vi "Charging_Find IPG MICS IDs.vi"(6 "error in":errorcluster, 8 "MICS_Config_In":T1={"ConfigFlags"=0, "ImplantID"=0, "CompanyID"=187, "Normal_Comm"={"RF_Channel"=4, "UserData"=0, "TX_Mod"=0, "RX_Mod"=0, "RX_BlockSize"=15, "BlockPerPack"=31, "TX_BlockSize"=15}, "Emerg_Comm"={"RF_Channel"=4, "UserData"=0, "TX_Mod"=0, "RX_Mod"=0, "TX_BlockSize"=15, "BlockPerPack"=31, "RX_BlockSize"=15}, "ImplantRev"=4, "245TX_PowerCal"=0, "245TX_Power"=10, "CCA_RSSI_Thresholds"={"ch0"=2650, "ch1"=2650, "ch2"=2650, "ch3"=2650, "ch4"=2650, "ch5"=2650, "ch6"=2650, "ch7"=2650, "ch8"=2650, "ch9"=2650}} {"ImplantID" format="%04x"; "CompanyID" format="%.0x"; "Normal_Comm"."RF_Channel" items=["0", "1", "2", "3", "4", "5", "6", "7", "8", "9"]; "Normal_Comm"."UserData" items=["0 - 000"=0, "1 - 001"=16, "2 - 010"=32, "3 - 011"=48, "4 - 100"=64, "5 - 101"=80, "6 - 110"=96, "7 - 111"=112]; "Normal_Comm"."TX_Mod" items=["2FSK-FB"=0, "2FSK"=2, "4FSK"=3]; "Normal_Comm"."RX_Mod" items=["2FSK-FB"=0, "2FSK"=8, "4FSK"=12]; "Normal_Comm"."RX_BlockSize" items=["2"=2, "3"=3, "4"=4, "5"=5, "6"=6, "7"=7, "8"=8, "9"=9, "10"=10, "11"=11, "12"=12, "13"=13, "14"=14, "15"=15, "16"=16, "17"=17, "18"=18, "19"=19, "20"=20, "21"=21, "22"=22, "23"=23, "24"=24, "25"=25, "26"=26, "27"=27, "28"=28, "29"=29, "30"=30, "31"=31]; "Normal_Comm"."BlockPerPack" items=["1"=1, "2"=2, "3"=3, "4"=4, "5"=5, "6"=6, "7"=7, "8"=8, "9"=9, "10"=10, "11"=11, "12"=12, "13"=13, "14"=14, "15"=15, "16"=16, "17"=17, "18"=18, "19"=19, "20"=20, "21"=21, "22"=22, "23"=23, "24"=24, "25"=25, "26"=26, "27"=27, "28"=28, "29"=29, "30"=30, "31"=31]; "Normal_Comm"."TX_BlockSize" items=["2"=2, "3"=3, "4"=4, "5"=5, "6"=6, "7"=7, "8"=8, "9"=9, "10"=10, "11"=11, "12"=12, "13"=13, "14"=14, "15"=15, "16"=16, "17"=17, "18"=18, "19"=19, "20"=20, "21"=21, "22"=22, "23"=23, "24"=24, "25"=25, "26"=26, "27"=27, "28"=28, "29"=29, "30"=30, "31"=31]; "Emerg_Comm"."RF_Channel" items=["0", "1", "2", "3", "4", "5", "6", "7", "8", "9"]; "Emerg_Comm"."UserData" items=["0 - 000"=0, "1 - 001"=16, "2 - 010"=32, "3 - 011"=48, "4 - 100"=64, "5 - 101"=80, "6 - 110"=96, "7 - 111"=112]; "Emerg_Comm"."TX_Mod" items=["2FSK-FB"=0, "2FSK"=2, "4FSK"=3]; "Emerg_Comm"."RX_Mod" items=["2FSK-FB"=0, "2FSK"=8, "4FSK"=12]; "Emerg_Comm"."TX_BlockSize" items=["2"=2, "3"=3, "4"=4, "5"=5, "6"=6, "7"=7, "8"=8, "9"=9, "10"=10, "11"=11, "12"=12, "13"=13, "14"=14, "15"=15, "16"=16, "17"=17, "18"=18, "19"=19, "20"=20, "21"=21, "22"=22, "23"=23, "24"=24, "25"=25, "26"=26, "27"=27, "28"=28, "29"=29, "30"=30, "31"=31]; "Emerg_Comm"."BlockPerPack" items=["1"=1, "2"=2, "3"=3, "4"=4, "5"=5, "6"=6, "7"=7, "8"=8, "9"=9, "10"=10, "11"=11, "12"=12, "13"=13, "14"=14, "15"=15, "16"=16, "17"=17, "18"=18, "19"=19, "20"=20, "21"=21, "22"=22, "23"=23, "24"=24, "25"=25, "26"=26, "27"=27, "28"=28, "29"=29, "30"=30, "31"=31]; "Emerg_Comm"."RX_BlockSize" items=["2"=2, "3"=3, "4"=4, "5"=5, "6"=6, "7"=7, "8"=8, "9"=9, "10"=10, "11"=11, "12"=12, "13"=13, "14"=14, "15"=15, "16"=16, "17"=17, "18"=18, "19"=19, "20"=20, "21"=21, "22"=22, "23"=23, "24"=24, "25"=25, "26"=26, "27"=27, "28"=28, "29"=29, "30"=30, "31"=31]; "ImplantRev" items=["ZL70100"=0, "ZL70101"=1, "ZL70102"=4]; "245TX_PowerCal" items=["-29"=-29, "-4"=-4, "-2"=-2, "0"=0, "2"=2, "4"=4, "6"=6, "8"=8, "10"=10, "12"=12, "14"=14, "16"=16, "18"=18, "20"=20, "22"=22, "24"=24, "26"=26, "27"=27]; "245TX_Power" items=["-29"=-29, "-4"=-4, "-2"=-2, "0"=0, "2"=2, "4"=4, "6"=6, "8"=8, "10"=10, "12"=12, "14"=14, "16"=16, "18"=18, "20"=20, "22"=22, "24"=24, "26"=26, "27"=27]}, 9 "MICS COM port":refnum<visa-resource-name>="COM11") -> (0 "error out":errorcluster {"code" format="%.0x"}, 3 "detected MICS IDs":u32[](array[numeric]))   [LabVIEW 2020]
doc: "This function searches for IPGs MIC IDs. The MICS Setup and MICS Config operations are performed before searching for the MICS IDs."
panel:
  in  "Max # of Attempts to Find Device":i32=3
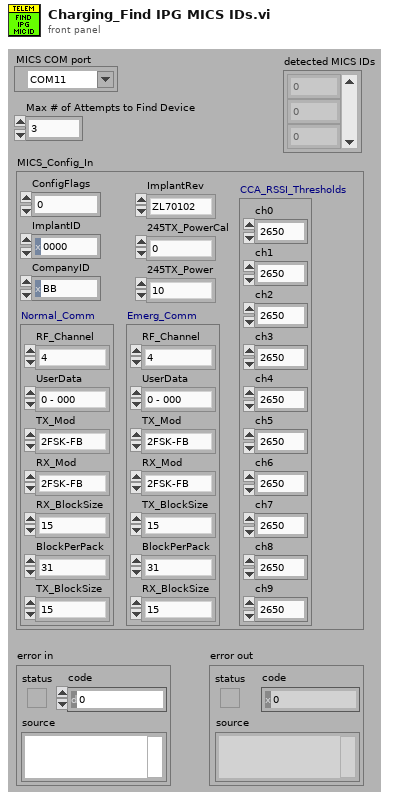
[diagram p1: front panel]
types:
  T1 = cluster{"ConfigFlags":u8, "ImplantID":u32, "CompanyID":u8, "Normal_Comm":cluster{"RF_Channel":u8, "UserData":u8, "TX_Mod":u8, "RX_Mod":u8, "RX_BlockSize":u8, "BlockPerPack":u8, "TX_BlockSize":u8}, "Emerg_Comm":cluster{"RF_Channel":u8, "UserData":u8, "TX_Mod":u8, "RX_Mod":u8, "TX_BlockSize":u8, "BlockPerPack":u8, "RX_BlockSize":u8}, "ImplantRev":u8, "245TX_PowerCal":i8, "245TX_Power":i8, "CCA_RSSI_Thresholds":cluster{"ch0":u16, "ch1":u16, "ch2":u16, "ch3":u16, "ch4":u16, "ch5":u16, "ch6":u16, "ch7":u16, "ch8":u16, "ch9":u16}}
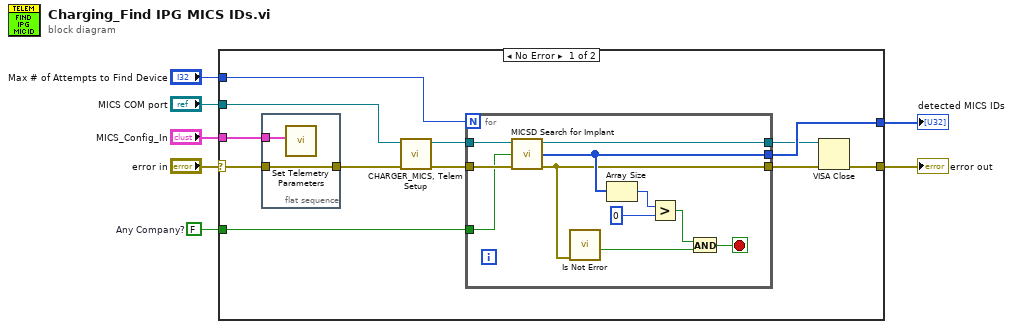
[diagram p0: block diagram]
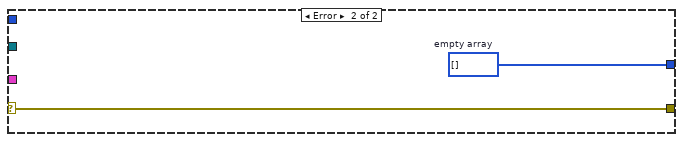
[diagram p2: hidden frame]
diagram:
  w6 = FALSE  # Any Company?
  n1 = case shown="No Error" "error in" {
    selector: "error in" -> [w9 w34]
    tunnel: "MICS COM port" -> [w16 _]
    tunnel: w6 -> [w15 _]
    tunnel: "MICS_Config_In" -> [w19 _]
    tunnel: [w17 w34] -> w3
    tunnel: [w18 w33] -> w2
    tunnel: "Max # of Attempts to Find Device" -> [w14 _]
    frame No Error {
      n2 = flat-sequence {
        tunnel: w19 -> [w21]
        tunnel: w9 -> [w20]
        tunnel: [w20] -> w8
        frame #0 {
          n3 = call "Set Telemetry Parameters.vi"("MICS_Config_In"=w21) -> ()  [unwired: 11 in]
        }
      }
      n4 = call "CHARGER_MICS, Telem Setup.vi"("error in"=w8, "VISA resource"=w16) -> ("error out"=w13:errorcluster, "VISA resource dup"=w12:refnum<visa-resource-name>)  [unwired: 8 in]
      n5 = for {
        N: w14 -> [_]
        tunnel: w13 -> [w32]
        tunnel: w12 -> [w31]
        tunnel: [w23] -> w11
        tunnel: [w30] -> w10
        tunnel: [w28] -> w18
        tunnel: w15 -> [w29]
        stop <- w24 stop-if-true
        n6 = call "MICSD Search for Implant.vi"("VISA Resource Name"=w31, "Any Company?(T)"=w29, "error in (no error)"=w32) -> ("dup VISA Resource Name"=w30:refnum<visa-resource-name>, "Detected MICS IDs"=w28:u32[], "error out"=w23:errorcluster)  [unwired: 9 in, 1 out]
        n7 = call "Is Not Error.vi"("error in"=w23) -> ("ready"=w22:bool)  [unwired: 5 in, 2 out]
        n8 = Array Size(array=w28) -> (size(s)=w27:i32)
        n9 = Greater?(x=w27, y=0) -> (0:w25:bool)
        n10 = And(x=w25, y=w22) -> (x .and. y?=w24:bool)
      }
      n11 = VISA Close(VISA resource name=w10, error in (no error)=w11) -> (error out=w17:errorcluster)
    }
    frame Error {
      w33 = u32[] []  # empty array
    }
  }
  "error out" <- w3
  "detected MICS IDs" <- w2
